vi "MainLogLoop.vi"(8 "error in (no error)":errorcluster, 10 "Sensors":T12={"Gyro"={"DevStatus"={"status"=FALSE, "code"=0, "source"=""}, "Analog Module"=enum."Controller 1", "Analog Channel"=enum."Invalid", "Offset"=0.0, "Gain (VoltsPerDegree/Second)"=0.0}, "Encoders"={"Left Drive CAN"={"DeviceStatus"={"status"=FALSE, "code"=0, "source"=""}, "Type"=enum."PWM", "PWM"={"Controller"=enum."Controller 1", "PWM Channel"=enum."PWM 1", "DeadBand"={"Name"="", "maxPositivePwm"=0, "minPositivePwm"=0, "centerPwm"=0, "maxNegativePwm"=0, "minNegativePwm"=0, "angularRange"=0}}, "CAN"={"Device Number"=0, "Control Mode"=enum."Percent VBus", "Semaphore"=refnum, "Max Vout"=12.0, "TalonSRX Control Mode"=enum."Percent VBus"}, "Invert"=FALSE, "TransformRef"=refnum, "InvTransformRef"=refnum}, "Right Drive CAN"={"DeviceStatus"={"status"=FALSE, "code"=0, "source"=""}, "Type"=enum."PWM", "PWM"={"Controller"=enum."Controller 1", "PWM Channel"=enum."PWM 1", "DeadBand"={"Name"="", "maxPositivePwm"=0, "minPositivePwm"=0, "centerPwm"=0, "maxNegativePwm"=0, "minNegativePwm"=0, "angularRange"=0}}, "CAN"={"Device Number"=0, "Control Mode"=enum."Percent VBus", "Semaphore"=refnum, "Max Vout"=12.0, "TalonSRX Control Mode"=enum."Percent VBus"}, "Invert"=FALSE, "TransformRef"=refnum, "InvTransformRef"=refnum}, "Strafe CAN"={"DeviceStatus"={"status"=FALSE, "code"=0, "source"=""}, "Type"=enum."PWM", "PWM"={"Controller"=enum."Controller 1", "PWM Channel"=enum."PWM 1", "DeadBand"={"Name"="", "maxPositivePwm"=0, "minPositivePwm"=0, "centerPwm"=0, "maxNegativePwm"=0, "minNegativePwm"=0, "angularRange"=0}}, "CAN"={"Device Number"=0, "Control Mode"=enum."Percent VBus", "Semaphore"=refnum, "Max Vout"=12.0, "TalonSRX Control Mode"=enum."Percent VBus"}, "Invert"=FALSE, "TransformRef"=refnum, "InvTransformRef"=refnum}, "Elevator CAN"={"DeviceStatus"={"status"=FALSE, "code"=0, "source"=""}, "Type"=enum."PWM", "PWM"={"Controller"=enum."Controller 1", "PWM Channel"=enum."PWM 1", "DeadBand"={"Name"="", "maxPositivePwm"=0, "minPositivePwm"=0, "centerPwm"=0, "maxNegativePwm"=0, "minNegativePwm"=0, "angularRange"=0}}, "CAN"={"Device Number"=0, "Control Mode"=enum."Percent VBus", "Semaphore"=refnum, "Max Vout"=12.0, "TalonSRX Control Mode"=enum."Percent VBus"}, "Invert"=FALSE, "TransformRef"=refnum, "InvTransformRef"=refnum}}, "Switches"={"Elevator Top"={"DevStatus"={"status"=FALSE, "code"=0, "source"=""}, "DIO Channel"=enum."DIO 1", "Controller"=enum."Controller 1", "CntIndex"=enum."Invalid", "Normally Closed"=FALSE}, "Elevator Bottom"={"DevStatus"={"status"=FALSE, "code"=0, "source"=""}, "DIO Channel"=enum."DIO 1", "Controller"=enum."Controller 1", "CntIndex"=enum."Invalid", "Normally Closed"=FALSE}, "Claw Outside"={"DevStatus"={"status"=FALSE, "code"=0, "source"=""}, "DIO Channel"=enum."DIO 1", "Controller"=enum."Controller 1", "CntIndex"=enum."Invalid", "Normally Closed"=FALSE}, "Tote Touch"={"DevStatus"={"status"=FALSE, "code"=0, "source"=""}, "DIO Channel"=enum."DIO 1", "Controller"=enum."Controller 1", "CntIndex"=enum."Invalid", "Normally Closed"=FALSE}}, "Arm Capper Pot"={"DevStatus"={"status"=FALSE, "code"=0, "source"=""}, "Controller"=enum."Controller 1", "Analog Channel"=enum."Invalid", "Invert Output"=FALSE}, "Arm Angle Pot"={"DevStatus"={"status"=FALSE, "code"=0, "source"=""}, "Controller"=enum."Controller 1", "Analog Channel"=enum."Invalid", "Invert Output"=FALSE}, "Sonar"={"Front"={"AIDeviceRef"={"DevStatus"={"status"=FALSE, "code"=0, "source"=""}, "Controller"=enum."Controller 1", "Analog Channel"=enum."Invalid"}, "Scaling factor (V/in)"=0.0098, "Average Bits"=3}, "Back"={"AIDeviceRef"={"DevStatus"={"status"=FALSE, "code"=0, "source"=""}, "Controller"=enum."Controller 1", "Analog Channel"=enum."Invalid"}, "Scaling factor (V/in)"=0.0098, "Average Bits"=3}}} {"Sonar"."Back"."Average Bits" max=15; "Sonar"."Front"."Average Bits" max=15}, 11 "Actuators":T1={"Drive"={"DevStatus"={"status"=FALSE, "code"=0, "source"=""}, "Motors[]"=[], "Square Inputs"=FALSE, "Max Output"=1.0}, "Strafe"={"DeviceStatus"={"status"=FALSE, "code"=0, "source"=""}, "Type"=enum."PWM", "PWM"={"Controller"=enum."Controller 1", "PWM Channel"=enum."Invalid", "DeadBand"={"Name"="", "maxPositivePwm"=0, "minPositivePwm"=0, "centerPwm"=0, "maxNegativePwm"=0, "minNegativePwm"=0, "angularRange"=0}}, "CAN"={"Device Number"=0, "Control Mode"=enum."Percent VBus", "Semaphore"=refnum, "Max Vout"=12.0, "TalonSRX Control Mode"=enum."Percent VBus"}, "Invert"=FALSE, "TransformRef"=refnum, "InvTransformRef"=refnum}, "Elevator Left"={"DeviceStatus"={"status"=FALSE, "code"=0, "source"=""}, "Type"=enum."PWM", "PWM"={"Controller"=enum."Controller 1", "PWM Channel"=enum."Invalid", "DeadBand"={"Name"="", "maxPositivePwm"=0, "minPositivePwm"=0, "centerPwm"=0, "maxNegativePwm"=0, "minNegativePwm"=0, "angularRange"=0}}, "CAN"={"Device Number"=0, "Control Mode"=enum."Percent VBus", "Semaphore"=refnum, "Max Vout"=12.0, "TalonSRX Control Mode"=enum."Percent VBus"}, "Invert"=FALSE, "TransformRef"=refnum, "InvTransformRef"=refnum}, "Elevator Right"={"DeviceStatus"={"status"=FALSE, "code"=0, "source"=""}, "Type"=enum."PWM", "PWM"={"Controller"=enum."Controller 1", "PWM Channel"=enum."Invalid", "DeadBand"={"Name"="", "maxPositivePwm"=0, "minPositivePwm"=0, "centerPwm"=0, "maxNegativePwm"=0, "minNegativePwm"=0, "angularRange"=0}}, "CAN"={"Device Number"=0, "Control Mode"=enum."Percent VBus", "Semaphore"=refnum, "Max Vout"=12.0, "TalonSRX Control Mode"=enum."Percent VBus"}, "Invert"=FALSE, "TransformRef"=refnum, "InvTransformRef"=refnum}, "Arm Clapper"={"DeviceStatus"={"status"=FALSE, "code"=0, "source"=""}, "Type"=enum."PWM", "PWM"={"Controller"=enum."Controller 1", "PWM Channel"=enum."Invalid", "DeadBand"={"Name"="", "maxPositivePwm"=0, "minPositivePwm"=0, "centerPwm"=0, "maxNegativePwm"=0, "minNegativePwm"=0, "angularRange"=0}}, "CAN"={"Device Number"=0, "Control Mode"=enum."Percent VBus", "Semaphore"=refnum, "Max Vout"=12.0, "TalonSRX Control Mode"=enum."Percent VBus"}, "Invert"=FALSE, "TransformRef"=refnum, "InvTransformRef"=refnum}, "Arm Angle"={"DeviceStatus"={"status"=FALSE, "code"=0, "source"=""}, "Type"=enum."PWM", "PWM"={"Controller"=enum."Controller 1", "PWM Channel"=enum."Invalid", "DeadBand"={"Name"="", "maxPositivePwm"=0, "minPositivePwm"=0, "centerPwm"=0, "maxNegativePwm"=0, "minNegativePwm"=0, "angularRange"=0}}, "CAN"={"Device Number"=0, "Control Mode"=enum."Percent VBus", "Semaphore"=refnum, "Max Vout"=12.0, "TalonSRX Control Mode"=enum."Percent VBus"}, "Invert"=FALSE, "TransformRef"=refnum, "InvTransformRef"=refnum}, "Arm Roller Left"={"DeviceStatus"={"status"=FALSE, "code"=0, "source"=""}, "Type"=enum."PWM", "PWM"={"Controller"=enum."Controller 1", "PWM Channel"=enum."Invalid", "DeadBand"={"Name"="", "maxPositivePwm"=0, "minPositivePwm"=0, "centerPwm"=0, "maxNegativePwm"=0, "minNegativePwm"=0, "angularRange"=0}}, "CAN"={"Device Number"=0, "Control Mode"=enum."Percent VBus", "Semaphore"=refnum, "Max Vout"=12.0, "TalonSRX Control Mode"=enum."Percent VBus"}, "Invert"=FALSE, "TransformRef"=refnum, "InvTransformRef"=refnum}, "Arm Roller Right"={"DeviceStatus"={"status"=FALSE, "code"=0, "source"=""}, "Type"=enum."PWM", "PWM"={"Controller"=enum."Controller 1", "PWM Channel"=enum."Invalid", "DeadBand"={"Name"="", "maxPositivePwm"=0, "minPositivePwm"=0, "centerPwm"=0, "maxNegativePwm"=0, "minNegativePwm"=0, "angularRange"=0}}, "CAN"={"Device Number"=0, "Control Mode"=enum."Percent VBus", "Semaphore"=refnum, "Max Vout"=12.0, "TalonSRX Control Mode"=enum."Percent VBus"}, "Invert"=FALSE, "TransformRef"=refnum, "InvTransformRef"=refnum}, "Wiper"={"DeviceStatus"={"status"=FALSE, "code"=0, "source"=""}, "Type"=enum."PWM", "PWM"={"Controller"=enum."Controller 1", "PWM Channel"=enum."Invalid", "DeadBand"={"Name"="", "maxPositivePwm"=0, "minPositivePwm"=0, "centerPwm"=0, "maxNegativePwm"=0, "minNegativePwm"=0, "angularRange"=0}}, "CAN"={"Device Number"=0, "Control Mode"=enum."Percent VBus", "Semaphore"=refnum, "Max Vout"=12.0, "TalonSRX Control Mode"=enum."Percent VBus"}, "Invert"=FALSE, "TransformRef"=refnum, "InvTransformRef"=refnum}}) -> (0 "error out":errorcluster)   [LabVIEW 2014]
uses:
  Utilities/Sensors.ctl
  <vilib>/Rock Robotics/WPI/Gyro/WPI_GyroDevRef.ctl
  <vilib>/Rock Robotics/SystemInterfaces/Typedef/FPGA_TypedefAnalogModule.ctl
  <vilib>/Rock Robotics/SystemInterfaces/AI/FPGA_AIChannel.ctl
  <vilib>/Rock Robotics/WPI/MotorControl/WPI_MotorControlDeviceRef.ctl
  <vilib>/Rock Robotics/WPI/MotorControl/WPI_MotorControlType.ctl
  <vilib>/Rock Robotics/SystemInterfaces/Typedef/FPGA_TypedefDigitalModule.ctl
  <vilib>/Rock Robotics/SystemInterfaces/DIO/FPGA_DIOPWMChannel.ctl
  <vilib>/Rock Robotics/WPI/PWM/WPI_PWMDeadband.ctl
  <vilib>/Rock Robotics/WPI/CAN/Jaguar/SubVIs/WPI_CANJaguar_ControlMode.ctl
  <vilib>/Rock Robotics/WPI/CAN/TalonSRX/WPI_CANTalonSRX_APIControlMode.ctl
  <vilib>/Rock Robotics/WPI/PWM/WPI_PWMTransform_ConPane.ctl
  <vilib>/Rock Robotics/WPI/Switch/WPI_SwitchDevRef.ctl
  <vilib>/Rock Robotics/SystemInterfaces/DIO/FPGA_DIOChannel.ctl
  <vilib>/Rock Robotics/SystemInterfaces/Counter/FPGA_CounterCtrSystemIndex.ctl
  <vilib>/Rock Robotics/WPI/Potentiometer/WPI_PotentiometerDevRef.ctl
  <vilib>/Rock Robotics/WPI/Ultrasonic/WPI_SonarMB1010AnalogDeviceRef.ctl
  <vilib>/Rock Robotics/WPI/AnalogChannel/WPI_AnalogChannelDevRef.ctl
  Utilities/Actuators.ctl
  <vilib>/Rock Robotics/WPI/RobotDrive/WPI_RobotDriveDevRef.ctl
  Utilities/Sensor Refname.ctl
  packet types.ctl
  <vilib>/Rock Robotics/WPI/DriverStation/WPI_DriverStationRobotMode2.ctl
  Utilities/Sensor Refname to String.vi
  <vilib>/Rock Robotics/Network Tables/SD Read Number.vi
  Main/Robot Global Data.vi
panel:
  out "result string to log":string
  # "Testing outputs:"
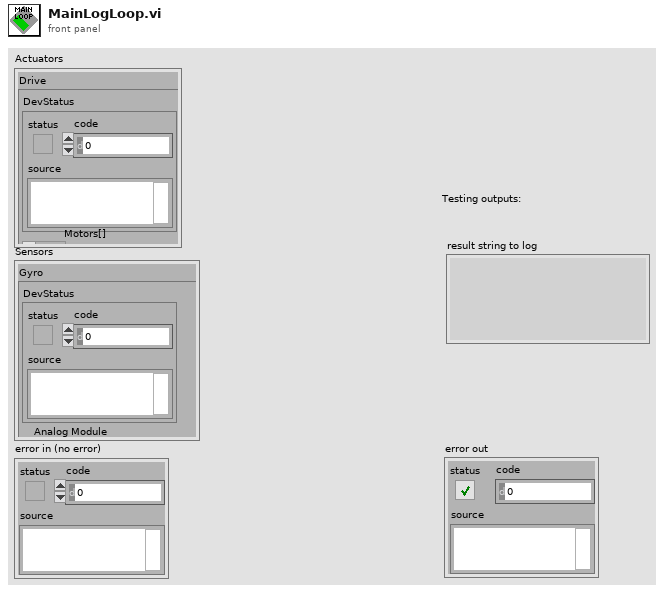
[diagram p1: front panel]
types:
  T1 = typedef "Actuators.ctl" = cluster{"Drive":T2, "Strafe":T3, "Elevator Left":T3, "Elevator Right":T3, "Arm Clapper":T3, "Arm Angle":T3, "Arm Roller Left":T3, "Arm Roller Right":T3, "Wiper":T3}
  T2 = typedef "WPI_RobotDriveDevRef.ctl" = cluster{"DevStatus":errorcluster, "Motors[]":T3[], "Square Inputs":bool, "Max Output":dbl}
  T3 = typedef "WPI_MotorControlDeviceRef.ctl" = cluster{"DeviceStatus":errorcluster, "Type":T4, "PWM":cluster{"Controller":T5, "PWM Channel":T6, "DeadBand":T7}, "CAN":cluster{"Device Number":u8, "Control Mode":T8, "Semaphore":T9, "Max Vout":dbl, "TalonSRX Control Mode":T10}, "Invert":bool, "TransformRef":T11, "InvTransformRef":T11}
  T4 = typedef "WPI_MotorControlType.ctl" = enum16{"PWM", "CAN", "CANTalonSRX"}
  T5 = typedef "FPGA_TypedefDigitalModule.ctl" = enum16{"Controller 1"}
  T6 = typedef "FPGA_DIOPWMChannel.ctl" = enum8{"PWM 0", "PWM 1", "PWM 2", "PWM 3", "PWM 4", "PWM 5", "PWM 6", "PWM 7", "PWM 8", "PWM 9", "PWM MXP 0", "PWM MXP 1", "PWM MXP 2", "PWM MXP 3", "PWM MXP 4", "PWM MXP 5", "PWM MXP 6", "PWM MXP 7", "PWM MXP 8", "PWM MXP 9", "Invalid"}
  T7 = typedef "WPI_PWMDeadband.ctl" = cluster{"Name":string, "maxPositivePwm":i32, "minPositivePwm":i32, "centerPwm":i32, "maxNegativePwm":i32, "minNegativePwm":i32, "angularRange":u16}
  T8 = typedef "WPI_CANJaguar_ControlMode.ctl" = enum8{"Percent VBus", "Current", "Speed", "Position", "Voltage"}
  T9 = typedef "Semaphore RefNum" = refnum<k1>
  T10 = typedef "WPI_CANTalonSRX_APIControlMode.ctl" = enum8{"Percent VBus", "Speed", "Position", "Slave", "Unchanged / Invalid"}
  T11 = typedef "WPI_PWMTransform_ConPane.ctl" = refnum<vi>
  T12 = typedef "Sensors.ctl" = cluster{"Gyro":T13, "Encoders":cluster{"Left Drive CAN":T3, "Right Drive CAN":T3, "Strafe CAN":T3, "Elevator CAN":T3}, "Switches":cluster{"Elevator Top":T16, "Elevator Bottom":T16, "Claw Outside":T16, "Tote Touch":T16}, "Arm Capper Pot":T19, "Arm Angle Pot":T19, "Sonar":cluster{"Front":T20, "Back":T20}}
  T13 = typedef "WPI_GyroDevRef.ctl" = cluster{"DevStatus":errorcluster, "Analog Module":T14, "Analog Channel":T15, "Offset":dbl, "Gain (VoltsPerDegree/Second)":dbl}
  T14 = typedef "FPGA_TypedefAnalogModule.ctl" = enum16{"Controller 1"}
  T15 = typedef "FPGA_AIChannel.ctl" = enum8{"AI 0", "AI 1", "AI 2", "AI 3", "AI MXP 0", "AI MXP 1", "AI MXP 2", "AI MXP 3", "Invalid"}
  T16 = typedef "WPI_SwitchDevRef.ctl" = cluster{"DevStatus":errorcluster, "DIO Channel":T17, "Controller":T5, "CntIndex":T18, "Normally Closed":bool}
  T17 = typedef "FPGA_DIOChannel.ctl" = enum8{"DIO 0", "DIO 1", "DIO 2", "DIO 3", "DIO 4", "DIO 5", "DIO 6", "DIO 7", "DIO 8", "DIO 9", "DIO MXP 0", "DIO MXP 1", "DIO MXP 2", "DIO MXP 3", "DIO MXP 4", "DIO MXP 5", "DIO MXP 6", "DIO MXP 7", "DIO MXP 8", "DIO MXP 9", "DIO MXP 10", "DIO MXP 11", "DIO MXP 12", "DIO MXP 13", "DIO MXP 14", "DIO MXP 15", "Invalid"}
  T18 = typedef "FPGA_CounterCtrSystemIndex.ctl" = enum8{"Ctr 0", "Ctr 1", "Ctr 2", "Ctr 3", "Ctr 4", "Ctr 5", "Ctr 6", "Ctr 7", "Invalid"}
  T19 = typedef "WPI_PotentiometerDevRef.ctl" = cluster{"DevStatus":errorcluster, "Controller":T14, "Analog Channel":T15, "Invert Output":bool}
  T20 = typedef "WPI_SonarMB1010AnalogDeviceRef.ctl" = cluster{"AIDeviceRef":T21, "Scaling factor (V/in)":dbl, "Average Bits":u8}
  T21 = typedef "WPI_AnalogChannelDevRef.ctl" = cluster{"DevStatus":errorcluster, "Controller":T14, "Analog Channel":T15}
  T22 = typedef "packet types.ctl" = enum16{"Log line", "Open File", "Send Header", "Set Time", "Send to LCD"}
  T23 = typedef "Sensor Refname.ctl" = enum16{"Gyro", "Elevator Top LS", "Elevator Bottom LS", "Claw Outside LS", "Left Drive Encoder", "Right Drive Encoder", "Strafe Encoder", "Elevator Encoder", "Ultrasonic Forward", "Ultrasonic Back", "Arm Angle POT", "Arm Clapper POT", "Accelerometer", "Tote LS", "DIP 1", "DIP 2", "DIP 3", "DIP 4"}
  T24 = typedef "WPI_SerialPortRef.ctl" = cluster{"DevStatus":errorcluster, "Serial Port Name":refnum<visa-resource-name>}
  T25 = cluster{"Left Drive CAN":T3, "Right Drive CAN":T3, "Strafe CAN":T3, "Elevator CAN":T3}
  T26 = typedef "WPI_AccelerometerDevRef.ctl" = cluster{"DevStatus":errorcluster, "Controller":T14, "Scaling":T27, "Analog Channels":T28, "I2C Bus":T29, "SPI Bus":T30, "Accel Range":T31, "ADXL345 Axes":T32, "Handle":i32, "Device Address":u8, "Accel Type":enum16{"Analog", "ADXL345 I2C", "ADXL345 SPI", "Internal"}}
  T27 = typedef "WPI_AccelerometerScaling.ctl" = cluster{"Gain (VoltsPerG)":dbl, "Center Voltage":dbl}
  T28 = typedef "WPI_AccelerometerAnalogChannels.ctl" = cluster{"X-Axis":T15, "Y-Axis":T15, "Z-Axis":T15}
  T29 = typedef "i2c_bus.ctl" = enum16{"I2C On-Board", "I2C MXP", "Invalid"}
  T30 = typedef "spi_bus.ctl" = enum16{"SPI On-Board, CS0", "SPI On-Board, CS1", "SPI On-Board, CS2", "SPI On-Board, CS3", "SPI MXP", "Invalid"}
  T31 = typedef "ADXL345 Range.ctl" = u8
  T32 = typedef "WPI_AccelerometerADXL345 Axes.ctl" = cluster{"X-Axis":bool, "Y-Axis":bool, "Z-Axis":bool}
  T33 = typedef "WPI_DriverStationRobotMode2.ctl" = enum16{"Autonomous Disabled", "Autonomous Enabled", "Teleop Disabled", "Teleop Enabled", "Disconnected", "Finish", "Test Disabled", "Test Enabled", "Emergency Stopped"}
  T34 = cluster{"X-Axis":dbl, "Y-Axis":dbl, "Z-Axis":dbl}
  T35 = typedef "WPI_CANTalonSRX_GlobalStatus.ctl" = cluster{"Applied Throttle":dbl, "Module Enabled":bool, "CAN Error":errorcluster, "Closed Loop Error":dbl, "Forward Limit Switch Closed":bool, "Reverse Limit Switch Closed":bool, "Sensor Position":dbl, "Sensor Velocity":dbl, "Current":dbl, "Sticky Fault - Over Temp":bool, "Sticky Fault - Under Voltage":bool, "Sticky Fault - Forward Limit":bool, "Sticky Fault - Reverse Limit":bool, "Sticky Fault - Forward Soft Limit":bool, "Sticky Fault - Reverse Soft Limit":bool, "Brake is Enabled":bool, "Encoder Position":dbl, "Encoder Velocity":dbl, "Encoder Index Count":dbl, "Encoder A Pin State":bool, "Encoder B Pin State":bool, "Encoder Index Pin State":bool, "Analog In":dbl, "Analog In Velocity":dbl, "Temperature (C)":dbl, "Battery Voltage":dbl}
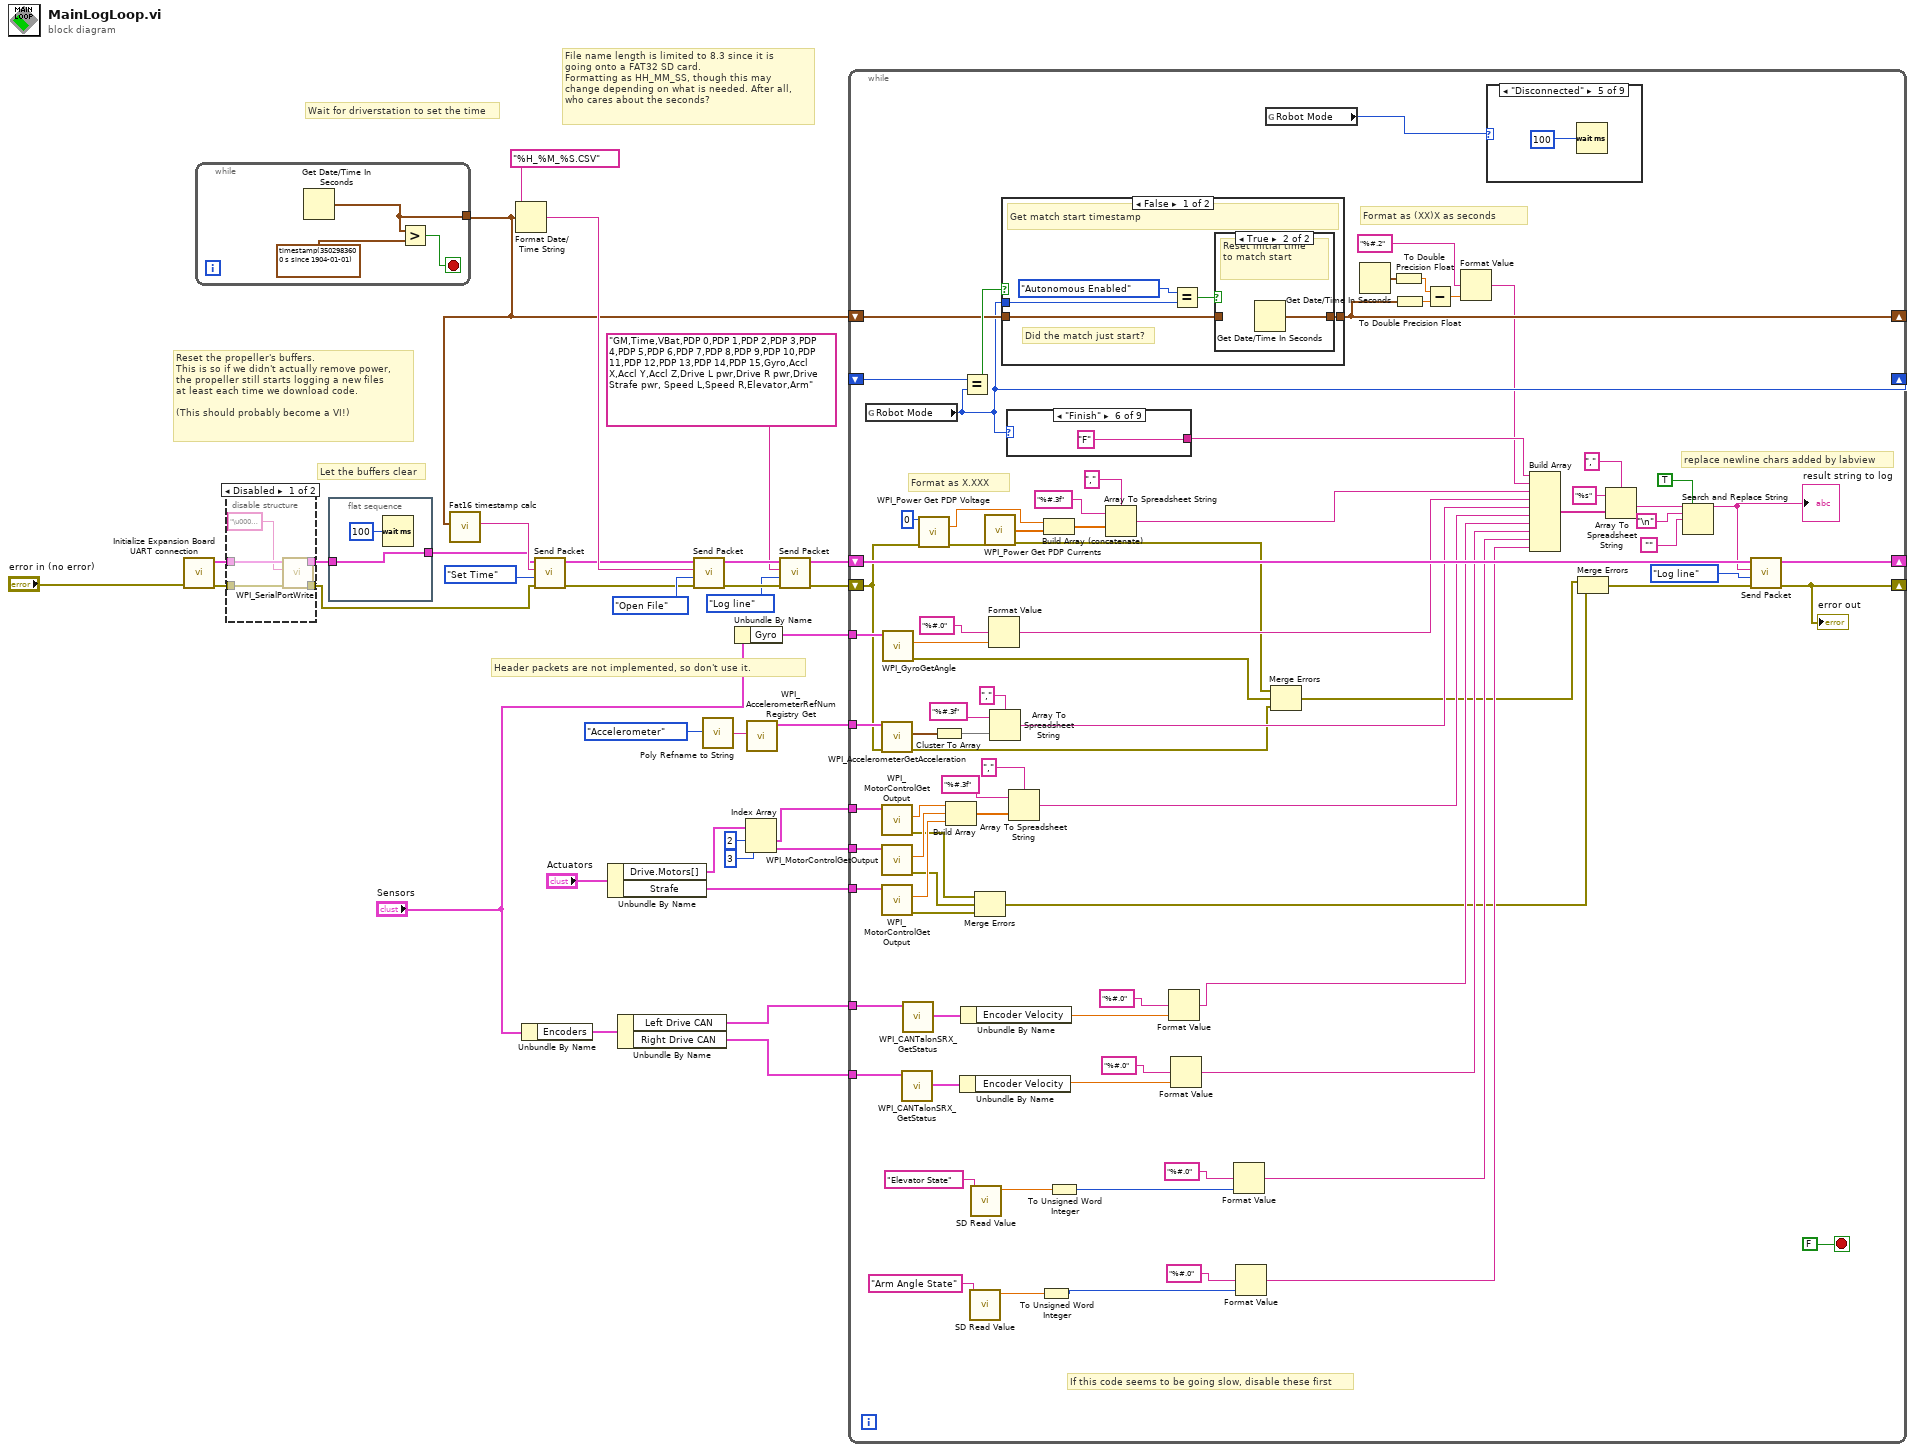
[diagram p0: block diagram]
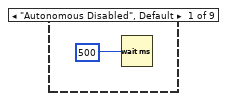
[diagram p3: hidden frame]
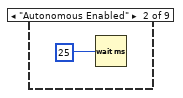
[diagram p4: hidden frame]
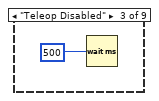
[diagram p5: hidden frame]
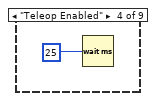
[diagram p6: hidden frame]
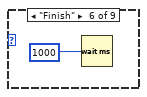
[diagram p7: hidden frame]
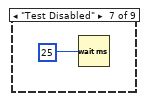
[diagram p8: hidden frame]
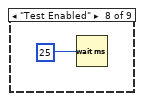
[diagram p9: hidden frame]
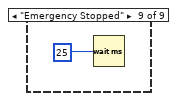
[diagram p10: hidden frame]
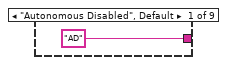
[diagram p13: hidden frame]
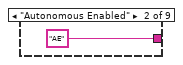
[diagram p14: hidden frame]
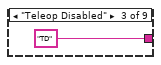
[diagram p15: hidden frame]
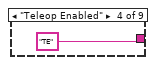
[diagram p16: hidden frame]
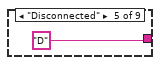
[diagram p17: hidden frame]
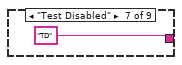
[diagram p18: hidden frame]
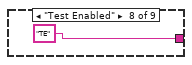
[diagram p19: hidden frame]
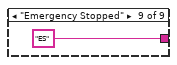
[diagram p20: hidden frame]
diagram:
  # "Let the buffers clear"
  # "Reset the propeller's buffers.\nThis is so if we didn't actually remove power,\nthe propeller still starts logging a new files \nat least each time we download code.\n\n(This should probably become a VI!)"
  # "File name length is limited to 8.3 since it is \ngoing onto a FAT32 SD card. \nFormatting as HH_MM_SS, though this may\nchange depending on what is needed. After all,\nwho cares about the seconds?"
  # "Wait for driverstation to set the time"
  # "Header packets are not implemented, so don't use it."
  n1 = call "Initialize Expansion Board UART connection.vi"("error in (no error)"="error in (no error)") -> ("error out"=w5:errorcluster, "SerialPortRef"=w4:T24)  [unwired: 9 in]
  n2 = while {
    tunnel: [w36] -> w7
    stop <- w37 stop-if-true
    n3 = Get Date/Time In Seconds() -> (seconds since 1Jan1904=w36:timestamp)
    n4 = Greater?(x=w36, y=timestamp(3502983600 s since 1904-01-01)) -> (0:w37:bool)
  }
  n5 = disable-structure shown="Disabled" {
    disable-tunnel: w5 -> [w43 w44]
    disable-tunnel: w4 -> [w42 w45]
    disable-tunnel: [w40 w45] -> w2
    disable-tunnel: [w39 w44] -> w1
    frame Disabled {
      n6 = call <vilib>:"WPI_SerialPortWrite.vi"("error in (no error)"=w43, "Buffer"="\u0004\u0004", "SerialPortRef"=w42) -> ("error out"=w39:errorcluster, "SerialPortRef"=w40:T24)  [unwired: 6 in, 1 out]
    }
    frame Enabled {
    }
  }
  n7 = flat-sequence {
    tunnel: [w47] -> w3
    tunnel: w2 -> [w47]
    frame #0 {
      n8 = Wait (ms)(milliseconds to wait=u32 100) -> ()  [unwired: 1 out]
    }
  }
  n9 = call "Fat16 timestamp calc.vi"("time stamp"=w7) -> ("timestamp as string"=w8:string)  [unwired: 10 in]
  n10 = Format Date/Time String(time format string (%c)="%H_%M_%S.CSV", seconds (now)=w7) -> (date/time string=w17:string)  [unwired: 1 in]
  n11 = Unbundle By Name("Sensors") -> ("Encoders"=w15:T25)
  n12 = call "Send Packet.vi"("error in (no error)"=w1, 7:packet_types."Set Time", "Log string"=w8, "SerialPortRef"=w3) -> ("error out"=w10:errorcluster, "SerialPortRef out"=w9:T24)  [unwired: 4 in]
  n13 = Unbundle By Name("Actuators") -> ("Drive.Motors[]"=w22:T3[], "Strafe"=w23:T3)
  n14 = Unbundle By Name(w15) -> ("Left Drive CAN"=w14:T3, "Right Drive CAN"=w13:T3)
  n15 = call "Send Packet.vi"("error in (no error)"=w10, 7:packet_types."Open File", "Log string"=w17, "SerialPortRef"=w9) -> ("error out"=w33:errorcluster, "SerialPortRef out"=w34:T24)  [unwired: 4 in]
  n16 = call-poly "Poly Refname to String.vi"("Sensor Refnames"=Sensor_Refname."Accelerometer" ("Sensor Refname")) -> ("Refname"=w29:string)
  n17 = Unbundle By Name("Sensors") -> ("Gyro"=w21:T13)
  n18 = Index Array(array=w22, index #1=2 ("index"), index #2=3 ("index")) -> (element #1=w27:T3, element #2=w26:T3)
  n19 = call <vilib>:"WPI_AccelerometerRefNum Registry Get.vi"("refnum name"=w29) -> ("AccelerometerDevRef"=w30:T26)  [unwired: 9 in, 1 out]
  n20 = call "Send Packet.vi"("error in (no error)"=w33, 7:packet_types."Log line", "Log string"="GM,Time,VBat,PDP 0,PDP 1,PDP 2,PDP 3,PDP 4,PDP 5,PDP 6,PDP 7,PDP 8,PDP 9,PDP 10,PDP 11,PDP 12,PDP 13,PDP 14,PDP 15,Gyro,Accl X,Accl Y,Accl Z,Drive L pwr,Drive R pwr,Drive Strafe pwr, Speed L,Speed R,Elevator,Arm", "SerialPortRef"=w34) -> ("error out"=w28:errorcluster, "SerialPortRef out"=w31:T24)  [unwired: 4 in]
  n21 = while {
    shift-right: [w81] -> _
    shift-left: w28 -> [w101]
    shift-right: [w130] -> _
    shift-left: w31 -> [w131]
    tunnel: w30 -> [w127]
    tunnel: w23 -> [w126]
    tunnel: w21 -> [w123]
    tunnel: w27 -> [w125]
    tunnel: w26 -> [w124]
    shift-right: [w119] -> _
    shift-left: _ -> [w122]
    shift-right: [w113] -> _
    shift-left: w7 -> [w120]
    tunnel: w14 -> [w93]
    tunnel: w13 -> [w94]
    stop <- FALSE stop-if-true
    # "If this code seems to be going slow, disable these first"
    # "replace newline chars added by labview"
    # "Format as (XX)X as seconds"
    # "Format as X.XXX"
    n22 = global read "Robot Global Data.vi" "Robot Mode"() -> (w119:T33)
    n23 = call <vilib>:"WPI_AccelerometerGetAcceleration.vi"("error in"=w101, "AccelerometerDevRef"=w127) -> ("error out"=w63:errorcluster, "Accelerations"=w66:T34)  [unwired: 7 in, 1 out]
    n24 = call <vilib>:"WPI_MotorControlGetOutput.vi"("MotorControlDevRef"=w125) -> ("error out"=w67:errorcluster, "Output"=w74:dbl)  [unwired: 8 in, 1 out]
    n25 = call <vilib>:"WPI_MotorControlGetOutput.vi"("MotorControlDevRef"=w124) -> ("error out"=w68:errorcluster, "Output"=w73:dbl)  [unwired: 8 in, 1 out]
    n26 = call <vilib>:"WPI_MotorControlGetOutput.vi"("MotorControlDevRef"=w126) -> ("error out"=w69:errorcluster, "Output"=w72:dbl)  [unwired: 8 in, 1 out]
    n27 = call <vilib>:"WPI_GyroGetAngle.vi"("GyroDevRef"=w123) -> ("error out"=w64:errorcluster, "Angle"=w77:dbl)  [unwired: 7 in, 2 out]
    n28 = call <vilib>:"WPI_CANTalonSRX_GetStatus.vi"("CAN Talon SRX Ref"=w94) -> ("Talon SRX Status"=w60:T35)  [unwired: 8 in, 2 out]
    n29 = call <vilib>:"WPI_CANTalonSRX_GetStatus.vi"("CAN Talon SRX Ref"=w93) -> ("Talon SRX Status"=w59:T35)  [unwired: 8 in, 2 out]
    n30 = call <vilib>:"WPI_Power Get PDP Voltage.vi"("Power Distribution Panel (0)"=u8 0, "error in"=w101) -> ("voltage (V)"=w110:dbl, "error out"=w102:errorcluster)  [unwired: 12 in]
    n31 = Cluster To Array(cluster=w66) -> (array=w65:dbl[])
    n32 = Build Array(w74, w73, w72) -> (w48:dbl[])
    n33 = Unbundle By Name(w60) -> ("Encoder Velocity"=w53:dbl)
    n34 = Unbundle By Name(w59) -> ("Encoder Velocity"=w55:dbl)
    n35 = Equal?(x=w122, y=w119) -> (x = y?=w121:bool)
    n36 = call-poly <vilib>:"SD Read Value.vi"("Name"="Arm Angle State") -> ("Numeric"=w58:dbl)  [unwired: 8 in, 2 out]
    n37 = call-poly <vilib>:"SD Read Value.vi"("Name"="Elevator State") -> ("Numeric"=w57:dbl)  [unwired: 8 in, 2 out]
    n38 = Merge Errors(w67, w68, w69) -> (w80:errorcluster)
    n39 = call <vilib>:"WPI_Power Get PDP Currents.vi"("error in"=w102) -> ("all currents (A)"=w100:dbl[], "error out"=w97:errorcluster)  [unwired: 12 in, 1 out]
    n40 = Format Value(format string="%#.0", value (0)=w77) -> (output string=w104:string)  [unwired: 1 in]
    n41 = Array To Spreadsheet String(delimiter (Tab)=",", array=w65, 3:"%#.3f" ("format string")) -> (spreadsheet string=w103:string)
    n42 = case shown="False" w121 {
      tunnel: w120 -> [w142 w148]
      tunnel: [w141 w148] -> w113
      tunnel: w119 -> [w145 _]
      frame False {
        # "Did the match just start?"
        # "Get match start timestamp"
        n43 = Equal?(x=WPI_DriverStationRobotMode2."Autonomous Enabled" ("Robot Mode"), y=w145) -> (x = y?=w143:bool)
        n44 = case shown="True" w143 {
          tunnel: w142 -> [w146 _]
          tunnel: [w146 w147] -> w141
          frame False {
            # "Match not starting,\ndo nothing"
          }
          frame True {
            # "Reset initial time\nto match start"
            n45 = Get Date/Time In Seconds() -> (seconds since 1Jan1904=w147:timestamp)
          }
        }
      }
      frame True {
        # "Wait until match starts"
      }
    }
    n46 = case shown="\"Finish\"" w119 {
      tunnel: ["AD" "AE" "TD" "TE" "D" "F" "TD" "TE" "ES"] -> w99
      frame "Autonomous Disabled", Default {
      }
      frame "Autonomous Enabled" {
      }
      frame "Teleop Disabled" {
      }
      frame "Teleop Enabled" {
      }
      frame "Disconnected" {
      }
      frame "Finish" {
      }
      frame "Test Disabled" {
      }
      frame "Test Enabled" {
      }
      frame "Emergency Stopped" {
      }
    }
    n47 = Array To Spreadsheet String(delimiter (Tab)=",", array=w48, 3:"%#.3f" ("format string")) -> (spreadsheet string=w87:string)
    n48 = To Unsigned Word Integer(number=w58) -> (unsigned 16bit integer=w49:u16)
    n49 = Build Array (concatenate)(w110, w100) -> (w109:dbl[])
    n50 = To Unsigned Word Integer(number=w57) -> (unsigned 16bit integer=w50:u16)
    n51 = Array To Spreadsheet String(delimiter (Tab)=",", array=w109, 3:"%#.3f" ("format string")) -> (spreadsheet string=w105:string)
    n52 = Format Value(format string="%#.0", value (0)=w55) -> (output string=w92:string)  [unwired: 1 in]
    n53 = Format Value(format string="%#.0", value (0)=w53) -> (output string=w91:string)  [unwired: 1 in]
    n54 = Format Value(format string="%#.0", value (0)=w50) -> (output string=w90:string)  [unwired: 1 in]
    n55 = Format Value(format string="%#.0", value (0)=w49) -> (output string=w89:string)  [unwired: 1 in]
    n56 = global read "Robot Global Data.vi" "Robot Mode"() -> (w95:T33)
    n57 = Merge Errors(w97, w64, w63) -> (w79:errorcluster)
    n58 = Get Date/Time In Seconds() -> (seconds since 1Jan1904=w116:timestamp)
    n59 = To Double Precision Float(number=w116) -> (double precision float=w115:dbl)
    n60 = To Double Precision Float(number=w113) -> (double precision float=w114:dbl)
    n61 = Subtract(x=w115, y=w114) -> (x-y=w117:dbl)
    n62 = Format Value(format string="%#.2", value (0)=w117) -> (output string=w98:string)  [unwired: 1 in]
    n63 = case shown="\"Disconnected\"" w95 {
      frame "Autonomous Disabled", Default {
        n64 = Wait (ms)(milliseconds to wait=u32 500) -> ()  [unwired: 1 out]
      }
      frame "Autonomous Enabled" {
        n65 = Wait (ms)(milliseconds to wait=u32 25) -> ()  [unwired: 1 out]
      }
      frame "Teleop Disabled" {
        n66 = Wait (ms)(milliseconds to wait=u32 500) -> ()  [unwired: 1 out]
      }
      frame "Teleop Enabled" {
        n67 = Wait (ms)(milliseconds to wait=u32 25) -> ()  [unwired: 1 out]
      }
      frame "Disconnected" {
        n68 = Wait (ms)(milliseconds to wait=u32 100) -> ()  [unwired: 1 out]
      }
      frame "Finish" {
        n69 = Wait (ms)(milliseconds to wait=u32 1000) -> ()  [unwired: 1 out]
      }
      frame "Test Disabled" {
        n70 = Wait (ms)(milliseconds to wait=u32 25) -> ()  [unwired: 1 out]
      }
      frame "Test Enabled" {
        n71 = Wait (ms)(milliseconds to wait=u32 25) -> ()  [unwired: 1 out]
      }
      frame "Emergency Stopped" {
        n72 = Wait (ms)(milliseconds to wait=u32 25) -> ()  [unwired: 1 out]
      }
    }
    n73 = Build Array(w99, w98, w105, w104, w103, w87, w92, w91, w90, w89) -> (w106:string[])
    n74 = Merge Errors(w79, w80) -> (w88:errorcluster)
    n75 = Array To Spreadsheet String(delimiter (Tab)=",", array=w106, 3:"%s" ("format string")) -> (spreadsheet string=w83:string)
    n76 = Search and Replace String(replace all?=TRUE ("replace all? (F)"), input string=w83, search string="\n", replace string="") -> (result string=w82:string)  [unwired: 4 in, 3 out]
    "result string to log" <- w82
    n77 = call "Send Packet.vi"("error in (no error)"=w88, 7:packet_types."Log line", "Log string"=w82, "SerialPortRef"=w131) -> ("error out"=w81:errorcluster, "SerialPortRef out"=w130:T24)  [unwired: 4 in]
    "error out" <- w81
  }
